vi "Resolve ID.vi"(8 "error in (no error)":errorcluster, 10 "Tag ID / Name":variant, 11 "Raw Message in":refnum<class "Raw Message.lvclass">) -> (0 "error out":errorcluster, 2 "Tag ID":u32, 3 "Raw Message out":refnum<class "Raw Message.lvclass">)   [LabVIEW 2020, in "Protobuf RAW.lvlib" / "Raw Message.lvclass"]
uses:
  Raw Message.lvclass
  Raw Message.lvclass/Raw Message.ctl
  <vilib>/Utility/Data Type/NI_Data Type.lvlib
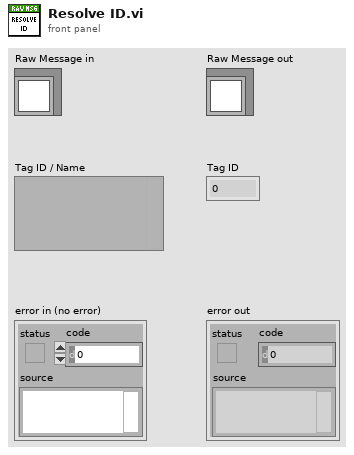
[diagram p1: front panel]
types:
  T1 = typedef "NI_Data Type.lvlib/Data Type.ctl" = enum8{"Invalid Type", "Void", "I8", "I16", "I32", "I64", "U8", "U16", "U32", "U64", "Single Float", "Double Float", "Extended Float", "Single Complex", "Double Complex", "Extended Complex", "Enum U8", "Enum U16", "Enum U32", "Enum U64", "Single Float With Unit", "Double Float With Unit", "Extended Float With Unit", "Single Complex with Unit", "Double Complex with Unit", "Extended Complex with Unit", "Boolean", "String", "Path", "Picture", "Tag", "Array", "Cluster", "Variant", "LV Variant", "Waveform", "Timestamp", "Digital Waveform", "Digital Data", "ExpressData", "Refnum", "External Data", "VI", "Poly VI", "LabVIEW Class Instance", "Fixed Point", "Set Collection", "Map Collection"}
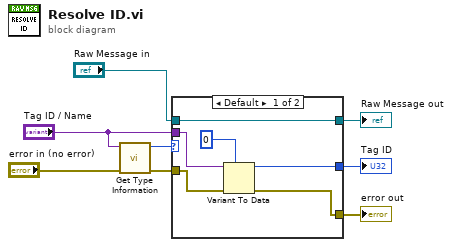
[diagram p0: block diagram]
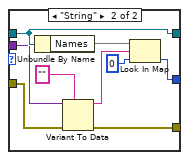
[diagram p2: hidden frame]
diagram:
  n1 = call <vilib>:"Get Type Information.vi"("error in (no error)"="error in (no error)", "variant"="Tag ID / Name") -> ("error out"=w4:errorcluster, "type"=w7:T1)  [unwired: 5 in, 3 out]
  n2 = case shown="Default" w7 {
    tunnel: "Raw Message in" -> [w9 w23]
    tunnel: [w9 w23] -> w5
    tunnel: w4 -> [w14 w21]
    tunnel: "Tag ID / Name" -> [w13 w20]
    tunnel: [w10 w17] -> w2
    tunnel: [w11 w15] -> w1
    frame Default {
      n3 = Variant To Data(error in=w14, type=u32 0 ("Tag ID"), Variant=w13) -> (data=w10:u32, error out=w11:errorcluster)
    }
    frame "String" {
      n4 = Unbundle By Name(w23) -> ("Names"=w22:map{string, u32})
      n5 = Variant To Data(error in=w21, type="", Variant=w20) -> (data=w18:string, error out=w15:errorcluster)
      n6 = Look In Map(map=w22, key=w18, default value=u32 0) -> (value=w17:u32)  [unwired: 1 out]
    }
  }
  "error out" <- w1
  "Raw Message out" <- w5
  "Tag ID" <- w2
